vi "Wire Matching Tunnels.vi"(2 "Error In":errorcluster, 3 "Case Refnum":refnum<vi>) -> (0 "error out":errorcluster, 1 "Case Refnum":refnum<vi>)   [LabVIEW 2012, in "Scripting Tools.lvlib"]
uses:
  <userlib>/_LAVAcr/Scripting Tools/Scripting Tools.lvlib
  <vilib>/Utility/VariantDataType/VariantType.lvlib
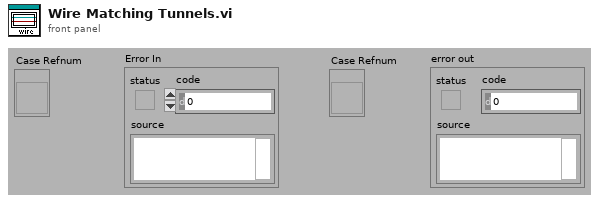
[diagram p1: front panel]
types:
  T1 = typedef "VariantType.lvlib/Type.ctl" = enum8{"Invalid Type", "Void", "I8", "I16", "I32", "I64", "U8", "U16", "U32", "U64", "Single Float", "Double Float", "Extended Float", "Single Complex", "Double Complex", "Extended Complex", "Enum U8", "Enum U16", "Enum U32", "Enum U64", "Single Float With Unit", "Double Float With Unit", "Extended Float With Unit", "Single Complex with Unit", "Double Complex with Unit", "Extended Complex with Unit", "Boolean", "String", "Path", "Picture", "Tag", "Array", "Cluster", "Variant", "LV Variant", "Waveform", "Timestamp", "Digital Waveform", "Digital Data", "ExpressData", "Refnum", "External Data", "VI", "Poly VI", "LabVIEW Class Instance", "Fixed Point"}
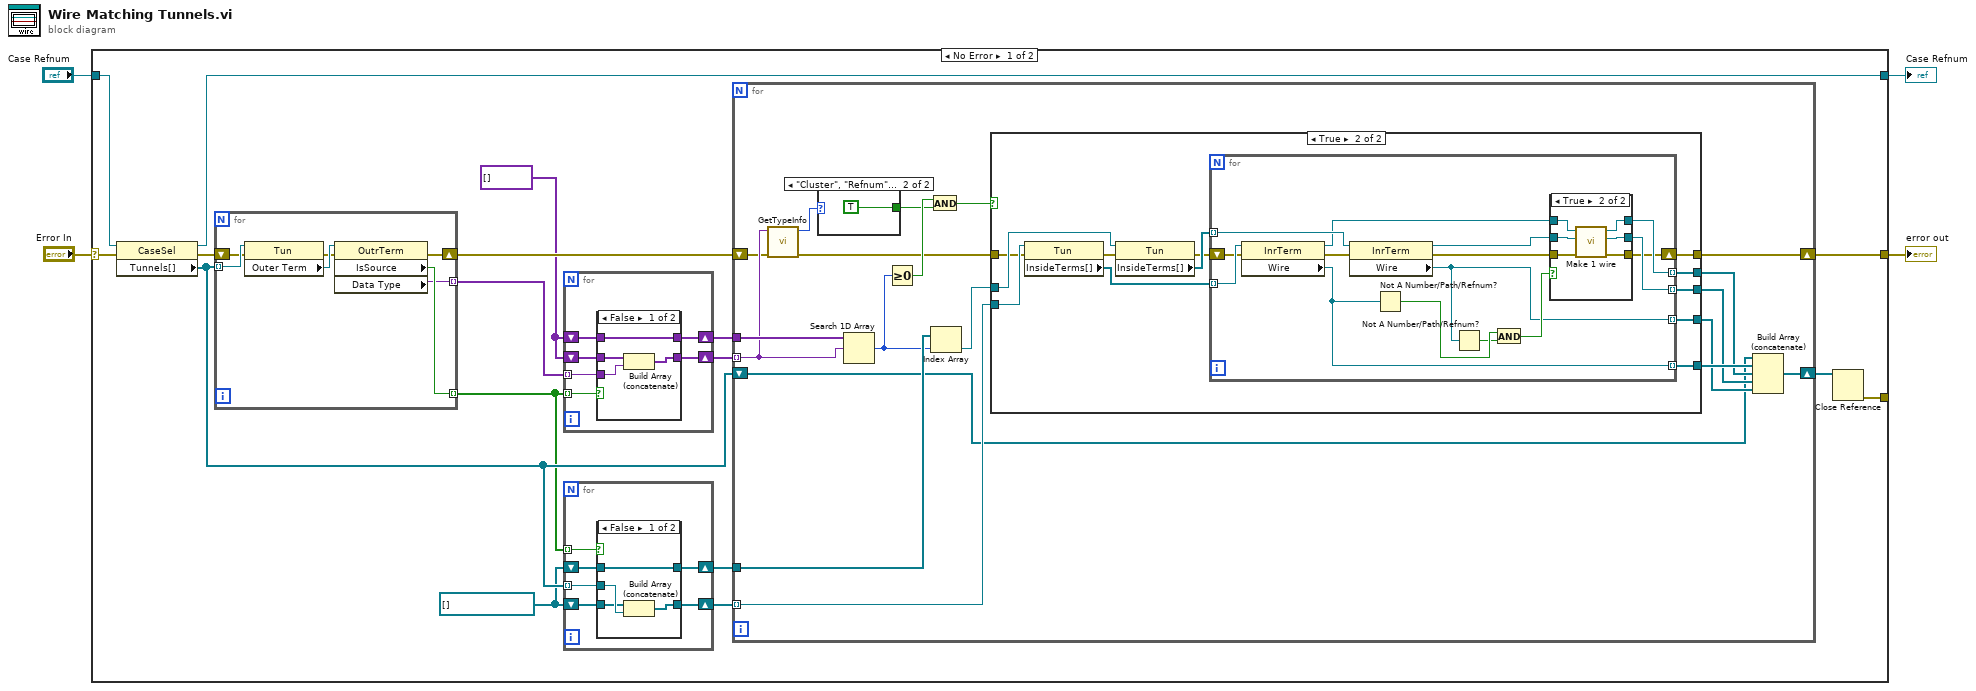
[diagram p0: block diagram]
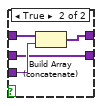
[diagram p2: hidden frame]
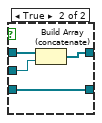
[diagram p3: hidden frame]
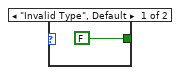
[diagram p6: hidden frame]
diagram:
  n1 = case shown="No Error" "Error In" {
    selector: "Error In" -> [w16 w116]
    tunnel: "Case Refnum" -> [w18 w115]
    tunnel: [w15 w116] -> w3
    tunnel: [w17 w115] -> w2
    tunnel: [w14 _] -> _
    frame No Error {
      w5 = variant[] []
      w6 = refnum<vi>[] []
      n2 = property class="CaseSel"(reference=w18, error in=w16) -> (reference out=w17:refnum<vi>, error out=w20:errorcluster, "Tunnels[]"=w13:refnum<vi>[])
      n3 = for {
        tunnel: w13 -> [w114] mode=indexing
        tunnel: [w111] -> w9 mode=indexing
        tunnel: [w110] -> w10 mode=indexing
        shift-right: [w109] -> w21
        shift-left: w20 -> [w108]
        n4 = property class="Tun"(reference=w114, error in=w108) -> (error out=w112:errorcluster, "Outer Term"=w113:refnum<vi>)  [unwired: 1 out]
        n5 = property class="OutrTerm"(reference=w113, error in=w112) -> (error out=w109:errorcluster, "IsSource"=w111:bool, "Data Type"=w110:variant)  [unwired: 1 out]
      }
      n6 = for {
        tunnel: w9 -> [w27] mode=indexing
        tunnel: w10 -> [w26] mode=indexing
        shift-right: [w25] -> w7
        shift-left: w5 -> [w24]
        shift-right: [w23] -> w8
        shift-left: w5 -> [w22]
        n7 = case shown="False" w27 {
          tunnel: w26 -> [w30 w35]
          tunnel: [w31 w34] -> w25
          tunnel: w24 -> [w31 w33]
          tunnel: [w29 w32] -> w23
          tunnel: w22 -> [w28 w32]
          frame False {
            n8 = Build Array (concatenate)(w28, w30) -> (w29:variant[])
          }
          frame True {
            n9 = Build Array (concatenate)(w33, w35) -> (w34:variant[])
          }
        }
      }
      n10 = for {
        tunnel: w9 -> [w41] mode=indexing
        tunnel: w13 -> [w40] mode=indexing
        shift-right: [w39] -> w11
        shift-left: w6 -> [w38]
        shift-right: [w37] -> w12
        shift-left: w6 -> [w36]
        n11 = case shown="False" w41 {
          tunnel: w40 -> [w44 w49]
          tunnel: [w45 w48] -> w39
          tunnel: w38 -> [w45 w47]
          tunnel: [w43 w46] -> w37
          tunnel: w36 -> [w42 w46]
          frame False {
            n12 = Build Array (concatenate)(w42, w44) -> (w43:refnum<vi>[])
          }
          frame True {
            n13 = Build Array (concatenate)(w47, w49) -> (w48:refnum<vi>[])
          }
        }
      }
      n14 = for {
        tunnel: w8 -> [w64] mode=indexing
        tunnel: w7 -> [w68]
        tunnel: w11 -> [w67]
        tunnel: w12 -> [w59] mode=indexing
        shift-right: [w54] -> w19
        shift-left: w13 -> [w53]
        shift-right: [w50] -> w15
        shift-left: w21 -> [w52]
        n15 = call <vilib>:"GetTypeInfo.vi"("error in (no error)"=w52, "Variant"=w64) -> ("error out"=w51:errorcluster, "Type Enum"=w63:T1)  [unwired: 8 out]
        n16 = case shown="\"Cluster\", \"Refnum\", \"LabVIEW Class Instance\"" w63 {
          tunnel: [FALSE TRUE] -> w62
          frame "Invalid Type", Default {
          }
          frame "Cluster", "Refnum", "LabVIEW Class Instance" {
          }
        }
        n17 = Search 1D Array(1D array=w68, element=w64) -> (index of element=w66:i32)  [unwired: 1 out]
        n18 = Greater Or Equal To 0?(x=w66) -> (x >= 0?=w65:bool)
        n19 = And(x=w65, y=w62) -> (x .and. y?=w61:bool)
        n20 = Index Array(array=w67, index=w66) -> (element=w60:refnum<vi>)
        n21 = case shown="True" w61 {
          tunnel: w60 -> [_ w80]
          tunnel: w59 -> [_ w81]
          tunnel: [_ w77] -> w57
          tunnel: [_ w76] -> w56
          tunnel: [_ w75] -> w58
          tunnel: [_ w74] -> w55
          tunnel: w51 -> [w69 w73]
          tunnel: [w69 w70] -> w50
          frame False {
          }
          frame True {
            n22 = property class="Tun"(reference=w81, error in=w73) -> (error out=w72:errorcluster, "InsideTerms[]"=w79:refnum<vi>[])  [unwired: 1 out]
            n23 = property class="Tun"(reference=w80, error in=w72) -> (error out=w71:errorcluster, "InsideTerms[]"=w78:refnum<vi>[])  [unwired: 1 out]
            n24 = for {
              tunnel: w79 -> [w96] mode=indexing
              tunnel: w78 -> [w95] mode=indexing
              tunnel: [w89] -> w77 mode=indexing
              tunnel: [w88] -> w76 mode=indexing
              tunnel: [w87] -> w75 mode=indexing
              tunnel: [w86] -> w74 mode=indexing
              shift-right: [w82] -> w70
              shift-left: w71 -> [w85]
              n25 = property class="InrTerm"(reference=w96, error in=w85) -> (reference out=w91:refnum<vi>, error out=w84:errorcluster, "Wire"=w87:refnum<vi>)
              n26 = property class="InrTerm"(reference=w95, error in=w84) -> (reference out=w90:refnum<vi>, error out=w83:errorcluster, "Wire"=w86:refnum<vi>)
              n27 = Not A Number/Path/Refnum?(number/path/refnum=w87) -> (NaN/Path/Refnum?=w94:bool)
              n28 = Not A Number/Path/Refnum?(number/path/refnum=w86) -> (NaN/Path/Refnum?=w93:bool)
              n29 = And(x=w94, y=w93) -> (x .and. y?=w92:bool)
              n30 = case shown="True" w92 {
                tunnel: w91 -> [w99 w105]
                tunnel: w90 -> [w98 w104]
                tunnel: [w99 w103] -> w89
                tunnel: [w98 w102] -> w88
                tunnel: w83 -> [w97 w101]
                tunnel: [w97 w100] -> w82
                frame False {
                }
                frame True {
                  n31 = call "Make 1 wire.vi"("error in"=w101, "Wire Terminal 2"=w104, "Wire Terminal 1"=w105) -> ("error out"=w100:errorcluster, "Wire"=w102:refnum<vi>, "Wire Sink Terminal Out"=w103:refnum<vi>)  [unwired: 6 out]
                }
              }
            }
          }
        }
        n32 = Build Array (concatenate)(w53, w58, w57, w56, w55) -> (w54:refnum<vi>[])
      }
      n33 = Close Reference(reference=w19) -> (error out=w14:errorcluster)  [unwired: 1 in]
    }
    frame Error {
    }
  }
  "error out" <- w3
  "Case Refnum" <- w2
